vi "BM Filters.vi"(8 "error in (no error)":errorcluster, 11 "Bus Monitor in":refnum<class "Bus Monitor.lvclass">) -> (0 "error out":errorcluster, 3 "Bus Monitor out":refnum<class "Bus Monitor.lvclass">)   [LabVIEW 2020, in "Unit Tests.lvlib" / "Bus Monitor.lvclass"]
uses:
  Bus Monitor.lvclass
  Frames & Messages/TypeDefs/Command Type.ctl
  Bus Monitor/TypeDefs/Bus Monitor Configuration.ctl
  Bus Monitor/TypeDefs/Bus Monitor Timeout.ctl
  Bus Monitor/TypeDefs/Bus Monitor Timetag Behavior.ctl
  Bus Monitor/TypeDefs/Bus Monitor Record Requirement.ctl
  Bus Monitor/TypeDefs/Bus Monitor Timetag Configuration.ctl
  Bus Monitor.lvclass/Bus Monitor.ctl
  Filters/TypeDefs/Filter Configuration.ctl
  Frames & Messages/TypeDefs/Command Terminal Address.ctl
  Frames & Messages/TypeDefs/Command SubAddress.ctl
  Frames & Messages/TypeDefs/Simplified Parameter Data Table.ctl
  Frames & Messages/TypeDefs/Scaling Information.ctl
  Bus Monitor/Bus Monitor.lvclass
  C:/Users/MattJ/Desktop/git/bci-1553-labview-api/src/1553 SubComponent/1553 SubComponent.lvclass
  <vilib>/addons/_JKI Toolkits/Caraya/classes/Assert/Assert True.vi
  Filters/Filter/Filter.lvclass
  1553 Session/1553 Session.lvclass
  Dependencies/FPGA Interface/FPGA Interface.lvclass
  <vilib>/addons/_JKI Toolkits/Caraya/classes/Test/Test.lvclass
  BCI-1553 API.lvlib
  1553 Component/1553 Component.lvclass
  <vilib>/addons/_JKI Toolkits/Caraya/classes/Assert/Assert.lvclass
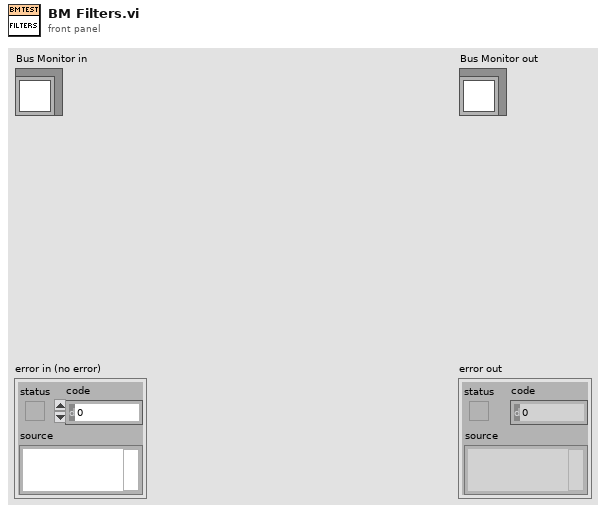
[diagram p1: front panel]
types:
  T1 = typedef "BCI-1553 API.lvlib/Bus Monitor.lvclass/Bus Monitor Record Requirement.ctl" = enum16{"Properly Encoded - Complete - Cmd Sync", "Properly Encoded - Complete - Cmd or Data Sync", "Properly Encoded Cmd Sync - At Least 2 Data Bits ", "Any Properly Encoded Sync - At Least 2 Data Bits"}
  T2 = typedef "BCI-1553 API.lvlib/Bus Monitor.lvclass/Bus Monitor Timetag Behavior.ctl" = enum16{"Last Bit of Last Word", "First Bit of Command Word", "Last Bit of Command Word", "Timetag Disabled"}
  T3 = typedef "BCI-1553 API.lvlib/Bus Monitor.lvclass/Bus Monitor Timeout.ctl" = enum16{"18us", "23us", "82us", "140us"}
  T4 = typedef "BCI-1553 API.lvlib/Bus Monitor.lvclass/Bus Monitor Configuration.ctl" = cluster{"Timeout":T3, "Gap Check":bool, "Timetag Behavior":T2, "Record Requirement":T1, "Cont Record After Inv Word":bool, "Ext Msg Flag Enable":bool, "48-bit Time Tag":bool, "Simple Mode":bool, "Bus Monitor Timetag Config":T5}
  T5 = typedef "BCI-1553 API.lvlib/Bus Monitor.lvclass/Bus Monitor Timetag Configuration.ctl" = enum16{"Disabled", "2us", "4us", "8us", "16us", "32us", "64us", "100ns"}
  T6 = typedef "BCI-1553 API.lvlib/Command Type.ctl" = enum16{"Transmit", "Receive"}
  T7 = typedef "BCI-1553 API.lvlib/Simplified Parameter Data Table.ctl" = cluster{"Parameter Name":string, "Base Word":u16, "Scaling Info":T8}
  T8 = typedef "BCI-1553 API.lvlib/Scaling Information.ctl" = cluster{"Bit Offset":i32, "Bit Count":i32, "LSB Resolution":dbl, "2's Complement":bool, "Big Endian":bool, "Sign Bit":bool}
  T9 = typedef "BCI-1553 API.lvlib/Filter Configuration.ctl" = cluster{"Filter Type":T6, "Terminal Address (0-30)":T10, "SubAddress (1-30)":T11, "Mode Code":bool, "Broadcast":bool, "RT-RT":bool, "Bus A":bool}
  T10 = typedef "BCI-1553 API.lvlib/Command Terminal Address.ctl" = enum16{"0", "1", "2", "3", "4", "5", "6", "7", "8", "9", "10", "11", "12", "13", "14", "15", "16", "17", "18", "19", "20", "21", "22", "23", "24", "25", "26", "27", "28", "29", "30", "Broadcast"}
  T11 = typedef "BCI-1553 API.lvlib/Command SubAddress.ctl" = enum16{"Mode Code", "1", "2", "3", "4", "5", "6", "7", "8", "9", "10", "11", "12", "13", "14", "15", "16", "17", "18", "19", "20", "21", "22", "23", "24", "25", "26", "27", "28", "29", "30"}
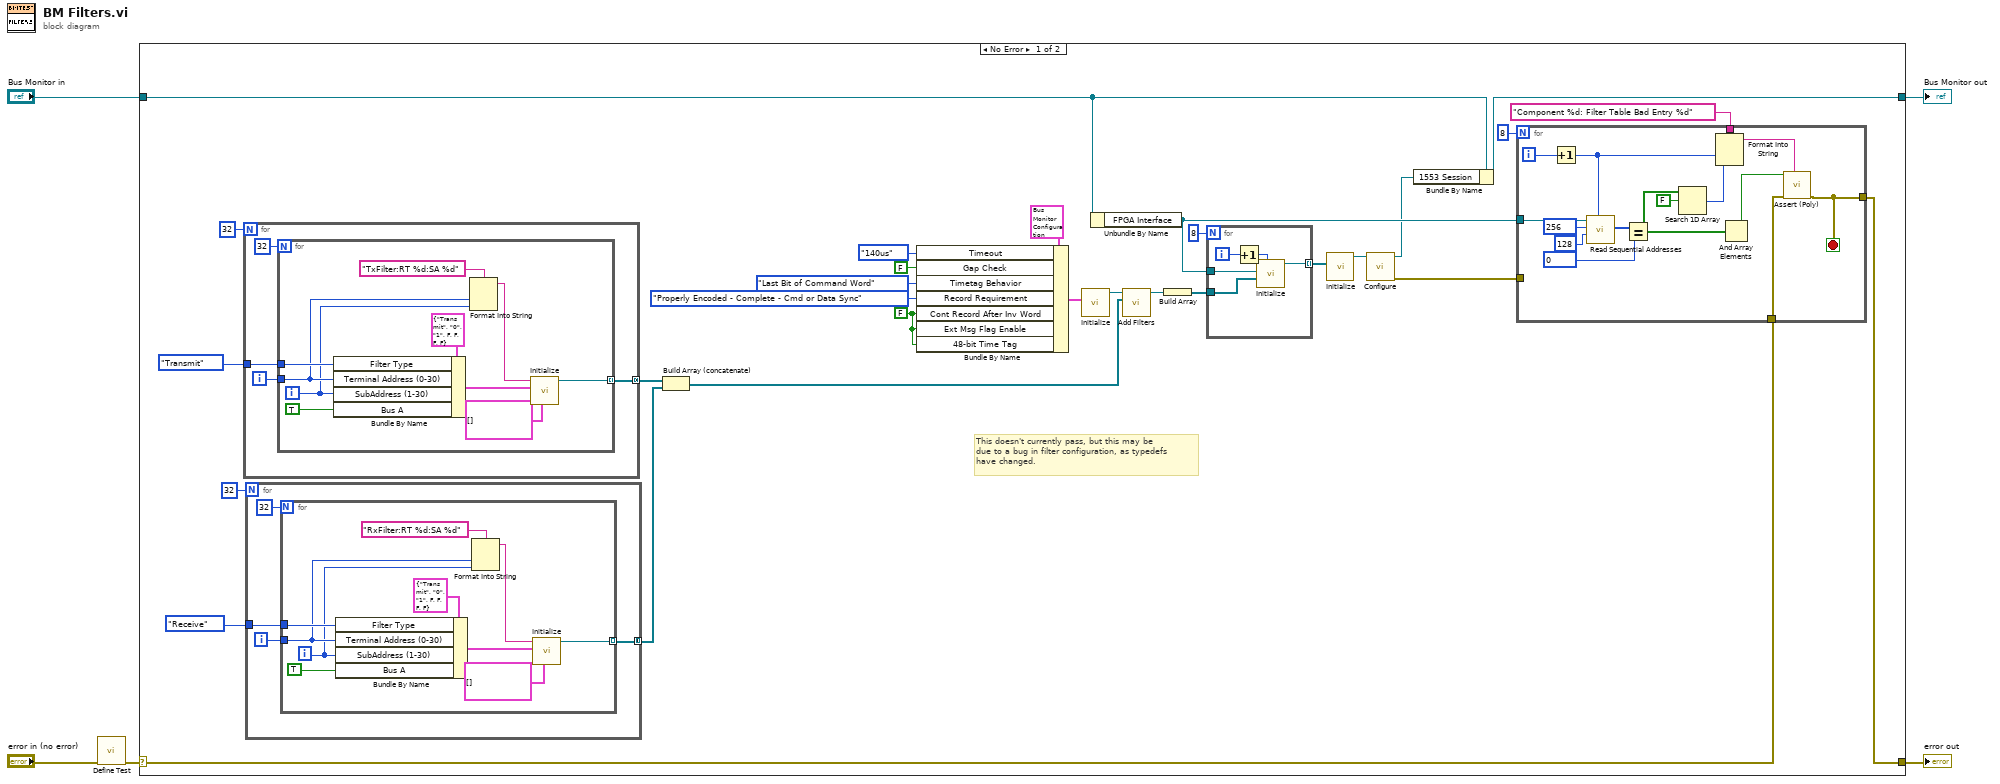
[diagram p0: block diagram]
diagram:
  n1 = call <vilib>:"Define Test.vi"("error in (no error)"="error in (no error)") -> ("error out"=w2:errorcluster)  [unwired: 9 in, 1 out]
  n2 = case shown="No Error" w2 {
    selector: w2 -> [w10 w84]
    tunnel: [w9 w84] -> w5
    tunnel: [w11 w83] -> w3
    tunnel: "Bus Monitor in" -> [w12 w83]
    frame No Error {
      w28 = FALSE ("Cont Record After Inv Word")
      # "This doesn't currently pass, but this may be \ndue to a bug in filter configuration, as typedefs\nhave changed."
      n3 = for {
        N: 32 -> [_]
        tunnel: Command_Type."Transmit" ("Filter Type") -> [w72]
        tunnel: [w69] -> w26 mode=concatenating
        i -> [w70]
        n4 = for {
          N: 32 -> [_]
          tunnel: w72 -> [w82]
          tunnel: w70 -> [w75]
          tunnel: [w80] -> w69 mode=indexing
          i -> [w73]
          n5 = Bundle By Name(cluster=T9 {"Filter Type"=enum."Transmit", "Terminal Address (0-30)"=enum."0", "SubAddress (1-30)"=enum."1", "Mode Code"=FALSE, "Broadcast"=FALSE, "RT-RT"=FALSE, "Bus A"=FALSE} ("Filter Configuration"), "Filter Type"=w82, "Terminal Address (0-30)"=w75, "SubAddress (1-30)"=w73, "Bus A"=TRUE) -> (w76:T9)
          n6 = Format Into String(format string="TxFilter:RT %d:SA %d", w75, w73) -> (resulting string=w78:string)  [unwired: 2 in, 1 out]
          n7 = call "Initialize.vi"("Parameters"=T7[] [], "Filter Configuration"=w76, "ID"=w78) -> ("Filter out"=w80:refnum<class "Filter.lvclass">)  [unwired: 7 in, 1 out]
        }
      }
      n8 = for {
        N: 32 -> [_]
        tunnel: Command_Type."Receive" ("Filter Type") -> [w58]
        tunnel: [w55] -> w25 mode=concatenating
        i -> [w56]
        n9 = for {
          N: 32 -> [_]
          tunnel: w58 -> [w68]
          tunnel: w56 -> [w63]
          tunnel: [w65] -> w55 mode=indexing
          i -> [w62]
          n10 = Bundle By Name(cluster=T9 {"Filter Type"=enum."Transmit", "Terminal Address (0-30)"=enum."0", "SubAddress (1-30)"=enum."1", "Mode Code"=FALSE, "Broadcast"=FALSE, "RT-RT"=FALSE, "Bus A"=FALSE} ("Filter Configuration"), "Filter Type"=w68, "Terminal Address (0-30)"=w63, "SubAddress (1-30)"=w62, "Bus A"=TRUE) -> (w66:T9)
          n11 = Format Into String(format string="RxFilter:RT %d:SA %d", w63, w62) -> (resulting string=w61:string)  [unwired: 2 in, 1 out]
          n12 = call "Initialize.vi"("Parameters"=T7[] [], "Filter Configuration"=w66, "ID"=w61) -> ("Filter out"=w65:refnum<class "Filter.lvclass">)  [unwired: 7 in, 1 out]
        }
      }
      n13 = Build Array (concatenate)(w26, w25) -> (w19:refnum<class "Filter.lvclass">[])
      n14 = Bundle By Name(cluster=T4 {"Timeout"=enum."18us", "Gap Check"=FALSE, "Timetag Behavior"=enum."Last Bit of Last Word", "Record Requirement"=enum."Properly Encoded - Complete - Cmd Sync", "Cont Record After Inv Word"=FALSE, "Ext Msg Flag Enable"=FALSE, "48-bit Time Tag"=FALSE, "Simple Mode"=FALSE, "Bus Monitor Timetag Config"=enum."Disabled"} ("Bus Monitor Configuration"), "Timeout"=Bus_Monitor_Timeout."140us", "Gap Check"=FALSE, "Timetag Behavior"=Bus_Monitor_Timetag_Behavior."Last Bit of Command Word", "Record Requirement"=Bus_Monitor_Record_Requirement."Properly Encoded - Complete - Cmd or Data Sync", "Cont Record After Inv Word"=w28, "Ext Msg Flag Enable"=w28, "48-bit Time Tag"=w28) -> (w27:T4)
      n15 = call "Initialize.vi"("Bus Monitor Configuration"=w27) -> ("Bus Monitor out"=w20:refnum<class "Bus Monitor.lvclass">)  [unwired: 9 in, 1 out]
      n16 = Unbundle By Name(w12) -> ("FPGA Interface"=w15:refnum<class "FPGA Interface.lvclass">)
      n17 = call-dynamic "Add Filters.vi"("Filters"=w19, "Bus Monitor in"=w20) -> ("Bus Monitor out"=w21:refnum<class "Bus Monitor.lvclass">)  [unwired: 8 in, 1 out]
      n18 = Build Array(w21) -> (w18:refnum<class "Bus Monitor.lvclass">[])
      n19 = for {
        N: 8 -> [_]
        tunnel: w15 -> [w52]
        tunnel: w18 -> [w51]
        tunnel: [w50] -> w17 mode=indexing
        i -> [w54]
        n20 = Increment(x=w54) -> (x+1=w53:i32)
        n21 = call "Initialize.vi"("Component ID (1-8)"=w53, "SubComponents"=w51, "FPGA Interface"=w52) -> ("1553 Component out"=w50:refnum<class "1553 Component.lvclass">)  [unwired: 7 in, 1 out]
      }
      n22 = call "Initialize.vi"("Components"=w17) -> ("1553 Board out"=w16:refnum<class "1553 Session.lvclass">)  [unwired: 9 in, 1 out]
      n23 = call-dynamic "Configure.vi"("1553 Board in"=w16) -> ("error out"=w14:errorcluster, "1553 Board out"=w13:refnum<class "1553 Session.lvclass">)  [unwired: 9 in]
      n24 = Bundle By Name(cluster=w12, "1553 Session"=w13) -> (w11:refnum<class "Bus Monitor.lvclass">)
      n25 = for {
        N: 8 -> [_]
        tunnel: w15 -> [w46]
        tunnel: [w36] -> w9
        tunnel: w10 -> [w37]
        tunnel: "Component %d: Filter Table Bad Entry %d" ("custom report message (\"\")") -> [w44]
        tunnel: w14 -> [_]
        i -> [w49]
        stop <- w36 stop-if-true
        n26 = Increment(x=w49) -> (x+1=w45:i32)
        n27 = call-dynamic "Read Sequential Addresses.vi"("Target IC (1-8)"=w45, "Addresses to Read"=u16 128, "Starting Address"=u16 256, "FPGA Interface in"=w46) -> ("Data"=w43:u16[])  [unwired: 6 in, 1 out]
        n28 = Equal?(x=w43, y=u16 0) -> (x = y?=w41:bool[])
        n29 = Search 1D Array(1D array=w41, element=FALSE) -> (index of element=w39:i32)  [unwired: 1 in]
        n30 = Format Into String(format string=w44, w45, w39) -> (resulting string=w35:string)  [unwired: 2 in, 1 out]
        n31 = And Array Elements(Boolean array=w41) -> (logical AND=w38:bool)
        n32 = call-poly <vilib>:"Assert (Poly).vi"("Label"=w35, "error in (no error)"=w37, "True?"=w38) -> ("error out"=w36:errorcluster)  [unwired: 7 in, 1 out]
      }
    }
    frame Error {
    }
  }
  "error out" <- w5
  "Bus Monitor out" <- w3
